vi "Run Tests (Path Array).vi"(7 "TextTestRunner in":refnum<class "TextTestRunner.lvclass">, 8 "error in (no error)":errorcluster, 10 "Test Paths":path[](array[path])) -> (0 "error out":errorcluster, 1 "test details":string, 2 "successful?":bool)   [LabVIEW 2011, in "VI Tester API.lvlib"]
doc: "Run test classes (TestCase or TestSuites) by file path. Test Paths are the file paths to the *.lvclass files on disk."
uses:
  VI Tester API.lvlib
  Classes/TextTestRunner/TextTestRunner.lvclass
  Libraries/VITesterUtilities.lvlib
panel:
  # "JKI VI Tester for LabVIEW\nhttp://jkisoft.com/vi-tester\nCopyright (C) 2007-2009, JKI <info@jkisoft.com>\nALL RIGHTS RESERVED"
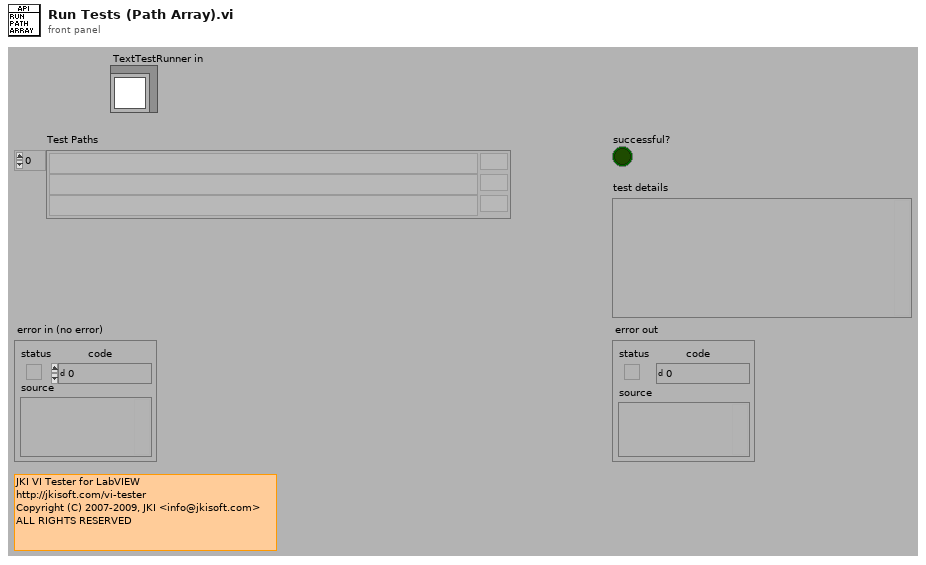
[diagram p1: front panel]
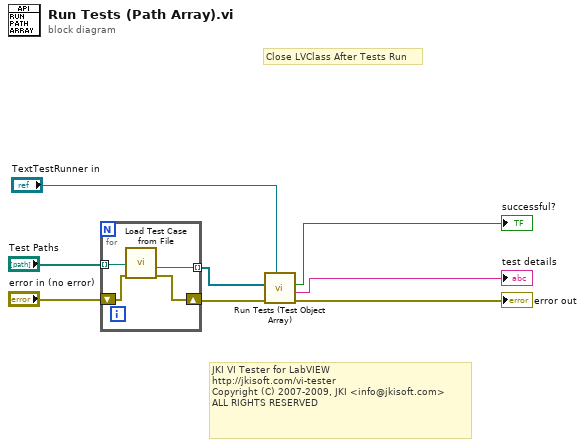
[diagram p0: block diagram]
diagram:
  # "JKI VI Tester for LabVIEW\nhttp://jkisoft.com/vi-tester\nCopyright (C) 2007-2009, JKI <info@jkisoft.com>\nALL RIGHTS RESERVED"
  # "Close LVClass After Tests Run"
  n1 = for {
    tunnel: [w10] -> w8 mode=indexing
    tunnel: "Test Paths" -> [w9] mode=indexing
    shift-right: [w11] -> w4
    shift-left: "error in (no error)" -> [w12]
    n2 = call "Load Test Case from File.vi"("error in"=w12, "Test Class Path"=w9) -> ("error out"=w11:errorcluster, "Test"=w10:refnum<class>)  [unwired: 8 in]
  }
  n3 = call "Run Tests (Test Object Array).vi"("TextTestRunner in"="TextTestRunner in", "error in (no error)"=w4, "Tests"=w8) -> ("error out"=→"error out":errorcluster, "test details"=→"test details":string, "successful?"=→"successful?":bool)  [unwired: 6 in]
